vi "Button Config Pane.vi"(6 "_SubPanelMessages":refnum<notifier>, 9 "_myEmbeddedToFrameEvent":T6, 10 "_myEmbedded.Exit":refnum<user-event>, 11 "_Property Bundle":cluster{"Name":string, "Value":variant}[](array[cluster])) -> (1 "_Connection Informations":T1, 2 "_Scripter Input":T8)   [LabVIEW 2021]
doc: "Reads the value from the user button on the NI myRIO."
uses:
  <vilib>/myRIO/Common/Express VI Framework/typedefs/Config Pane to Framework Ref.ctl
  <vilib>/myRIO/Common/Express VI Framework/typedefs/Data Validate Ref.ctl
  <vilib>/myRIO/Common/Express VI Framework/typedefs/Scripter Input.ctl
  <vilib>/myRIO/Common/Express VI Framework/typedefs/WireThrough Terminal Names.ctl
  <vilib>/myRIO/Common/Express VI Framework/typedefs/Instrument Driver Method Descriptor Array.ctl
  <vilib>/myRIO/Common/Express VI Framework/typedefs/Instrument Driver Method Descriptor.ctl
  <vilib>/myRIO/Common/Express VI Framework/typedefs/Sub Panel Messages.ctl
  <vilib>/myRIO/Express VI/Onboard Devices/Button/Button Images.ctl
  <vilib>/myRIO/Common/Express VI Framework/typedefs/Connection Informations.ctl
  <vilib>/myRIO/Common/Instrument Driver Framework/Utilities/typedefs/Channel Types.ctl
panel:
  out "Description":string
  out "_Button Location":T2
  in  "_Terminal Name \n(Edit and make value default)":string[](array[string])=["Value"]
  in  "_Default Alias String":string
  in  "_VI Default Name (Edit and make value default)":string="Button"
  in  "Name:":string caption="Node name:"
  in  "_WireThrough Info (Edit and make value default)":T3={"WireThrough Top In"="DIO Ref In", "WireThrough Bottom In"="error in (no error)", "WireThrough Top Out"="DIO Ref Out", "WireThrough Bottom Out"="error out"}
  in  "_Template Array (Edit and make value default)":T4=[{"Function Name"="Smart Open", "VI Path"=path "<vilib>/myRIO/Instrument Drivers/Onboard IO/DIO/vis", "Script"=TRUE, "Inputs"=[{"name"="Channel Names", "value"=variant, "Config Pane Only"=TRUE, "Build Array"=FALSE, "Bundle Cluster"=FALSE, "Show Term"=FALSE, "alias"=[], "Required Input"=FALSE}], "Outputs"=[], "VI Class"=enum."Open", "Controls Refs[]"=[], "Inline"=FALSE}, {"Function Name"="Open", "VI Path"=path "<vilib>/myRIO/Instrument Drivers/Onboard IO/DIO/vis", "Script"=FALSE, "Inputs"=[], "Outputs"=[], "VI Class"=enum."Open", "Controls Refs[]"=[], "Inline"=FALSE}, {"Function Name"="Read", "VI Path"=path "<vilib>/myRIO/Instrument Drivers/Onboard IO/DIO/vis", "Script"=TRUE, "Inputs"=[], "Outputs"=[{"name"="Values", "value"=variant, "Show Term"=TRUE, "Index Array"=TRUE, "Unbundle Cluster"=FALSE, "alias"=["Button"]}], "VI Class"=enum."Data", "Controls Refs[]"=[], "Inline"=FALSE}, {"Function Name"="Write", "VI Path"=path "<vilib>/myRIO/Instrument Drivers/Onboard IO/DIO/vis", "Script"=FALSE, "Inputs"=[{"name"="Values", "value"=variant, "Config Pane Only"=FALSE, "Build Array"=TRUE, "Bundle Cluster"=FALSE, "Show Term"=TRUE, "alias"=[], "Required Input"=FALSE}], "Outputs"=[], "VI Class"=enum."Data", "Controls Refs[]"=[], "Inline"=FALSE}, {"Function Name"="Close", "VI Path"=path "<vilib>/myRIO/Instrument Drivers/Onboard IO/DIO/vis", "Script"=FALSE, "Inputs"=[], "Outputs"=[], "VI Class"=enum."Close", "Controls Refs[]"=[], "Inline"=FALSE}]
  in  "_Test Close":bool
  # "User Visible Area"
  # "NOTE: Tab Order has been set\nfor this Front Panel.\n\nSee Edit>>Set Tabbing Order...\n\nAll controls that are not visible at \nruntime are excluded from Tabbing order\n\n\nTo exlude a control from context\nhelp prefix its label text with a '-'"
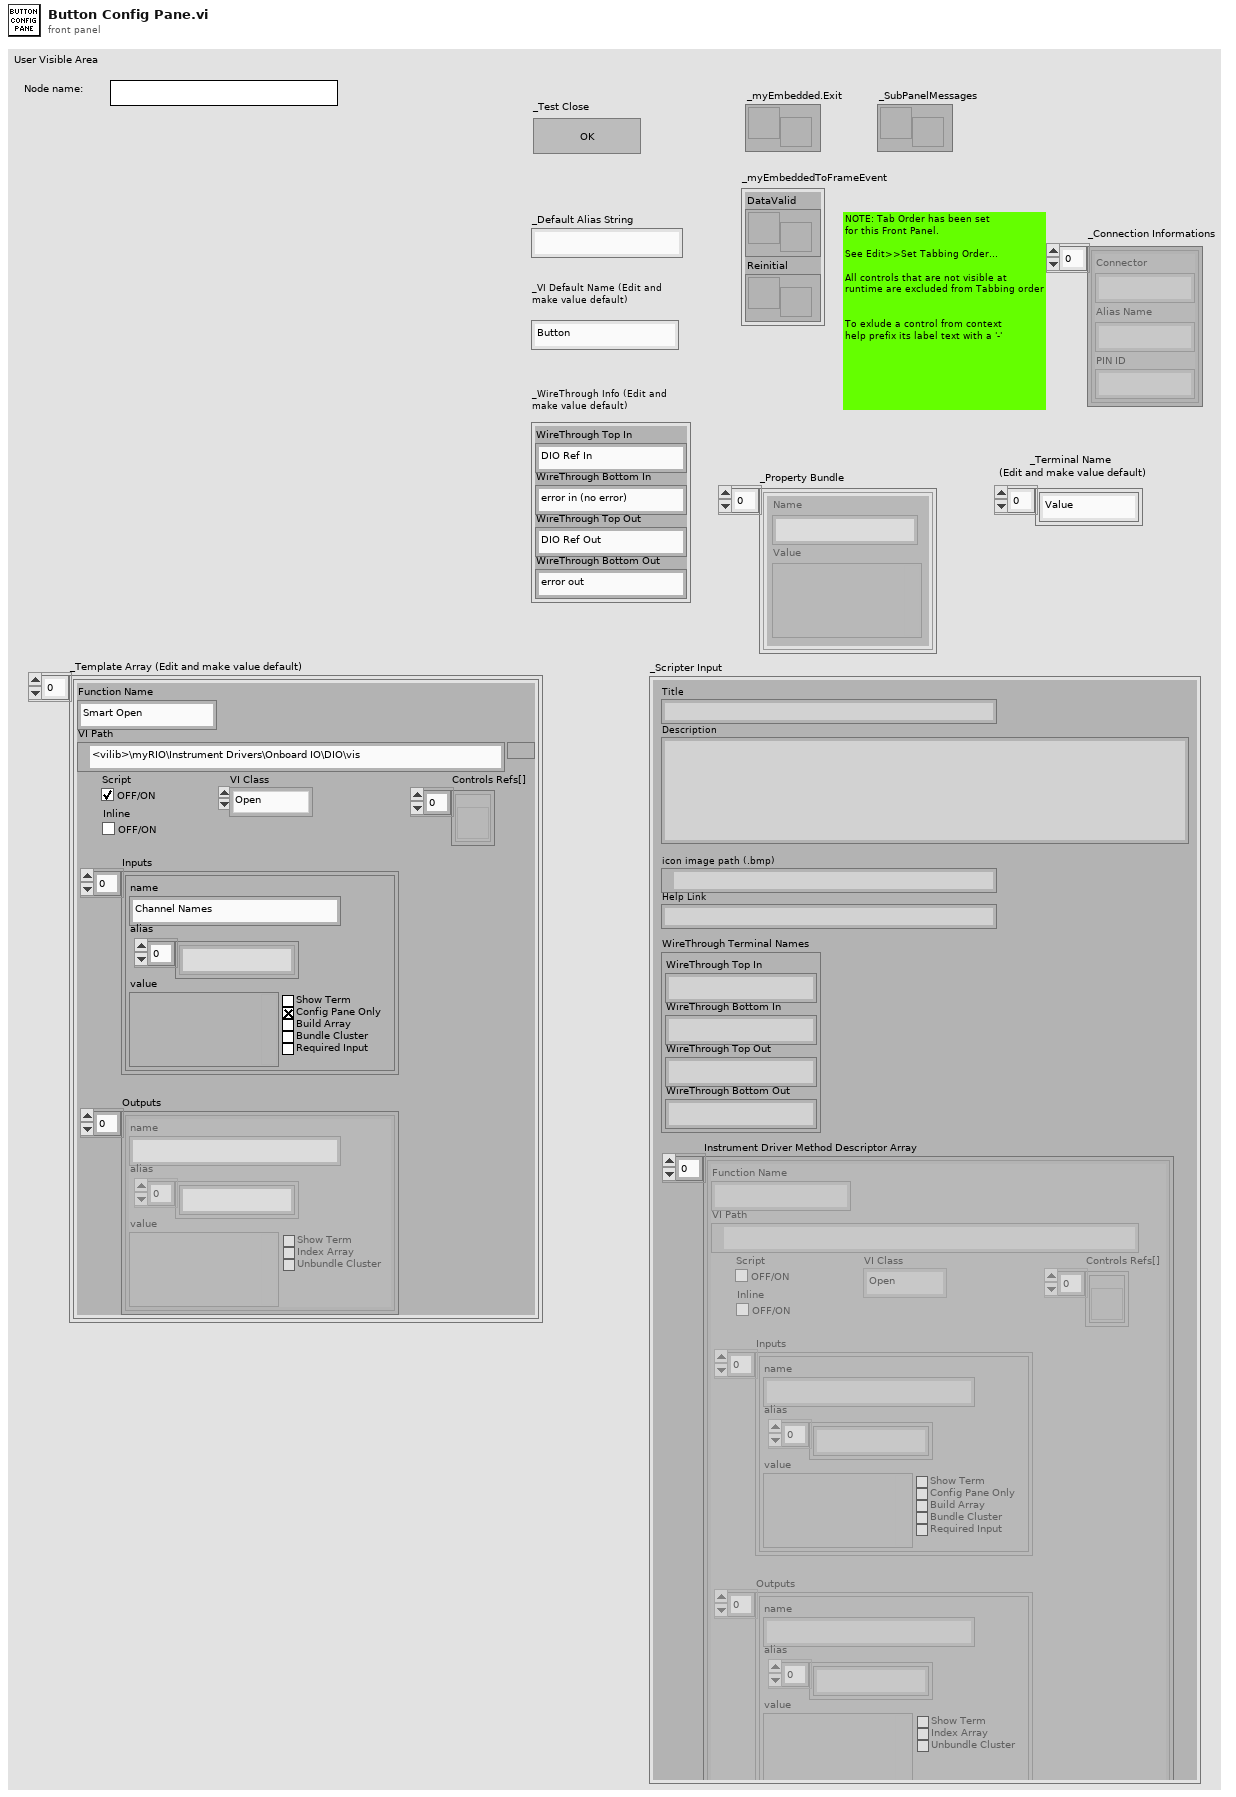
[diagram p1: front panel]
types:
  T1 = typedef "Connection Informations.ctl" = cluster{"Connector":string, "Alias Name":string, "PIN ID":string}[]
  T2 = typedef "Button Images.ctl" = u16
  T3 = typedef "WireThrough Terminal Names.ctl" = cluster{"WireThrough Top In":string, "WireThrough Bottom In":string, "WireThrough Top Out":string, "WireThrough Bottom Out":string}
  T4 = typedef "Instrument Driver Method Descriptor Array.ctl" = T5[]
  T5 = typedef "Instrument Driver Method Descriptor.ctl" = cluster{"Function Name":string, "VI Path":path, "Script":bool, "Inputs":cluster{"name":string, "value":variant, "Config Pane Only":bool, "Build Array":bool, "Bundle Cluster":bool, "Show Term":bool, "alias":string[], "Required Input":bool}[], "Outputs":cluster{"name":string, "value":variant, "Show Term":bool, "Index Array":bool, "Unbundle Cluster":bool, "alias":string[]}[], "VI Class":enum16{"Open", "Configure", "Data", "Manage", "Close"}, "Controls Refs[]":refnum<vi>[], "Inline":bool}
  T6 = typedef "Config Pane to Framework Ref.ctl" = cluster{"DataValid":T7, "Reinitial":refnum<user-event>}
  T7 = typedef "Data Validate Ref.ctl" = refnum<user-event>
  T8 = typedef "Scripter Input.ctl" = cluster{"Title":string, "Description":string, "icon image path (.bmp)":path, "Help Link":string, "WireThrough Terminal Names":T3, "Instrument Driver Method Descriptor Array":T4}
  T9 = typedef "Channel Types.ctl" = enum32{"Unknown", "AI", "AO", "DIO - DI", "DIO", "DIO - DO", "I2C", "PWM", "Encoder", "SPI", "UART", "Accelerometer", "DIO - LED", "DIO - Button", "AI (N Samples)", "AudioIn (N Samples)", "AO (N Samples)", "AudioOut (N Samples)", "DI (N Samples)", "DO (N Samples)", "AI IRQ", "DI IRQ", "Timer IRQ", "RSL", "Relay", "CAN", "AI (Continuous)", "AO (Continuous)"}
  T10 = typedef "Sub Panel Messages.ctl" = enum16{"Initialized"}
  T11 = typedef "Channel Info.ctl" = cluster{"Channel Name":string, "Alias":string, "Used?":bool, "Not Support?":bool, "Property Bundle":cluster{"Name":string, "Value":variant}[]}
  T12 = cluster{"name":string, "value":variant, "Config Pane Only":bool, "Build Array":bool, "Bundle Cluster":bool, "Show Term":bool, "alias":string[], "Required Input":bool}[]
  T13 = cluster{"name":string, "value":variant, "Config Pane Only":bool, "Build Array":bool, "Bundle Cluster":bool, "Show Term":bool, "alias":string[], "Required Input":bool}
  T14 = cluster{"name":string, "value":variant, "Show Term":bool, "Index Array":bool, "Unbundle Cluster":bool, "alias":string[]}[]
  T15 = cluster{"name":string, "value":variant, "Show Term":bool, "Index Array":bool, "Unbundle Cluster":bool, "alias":string[]}
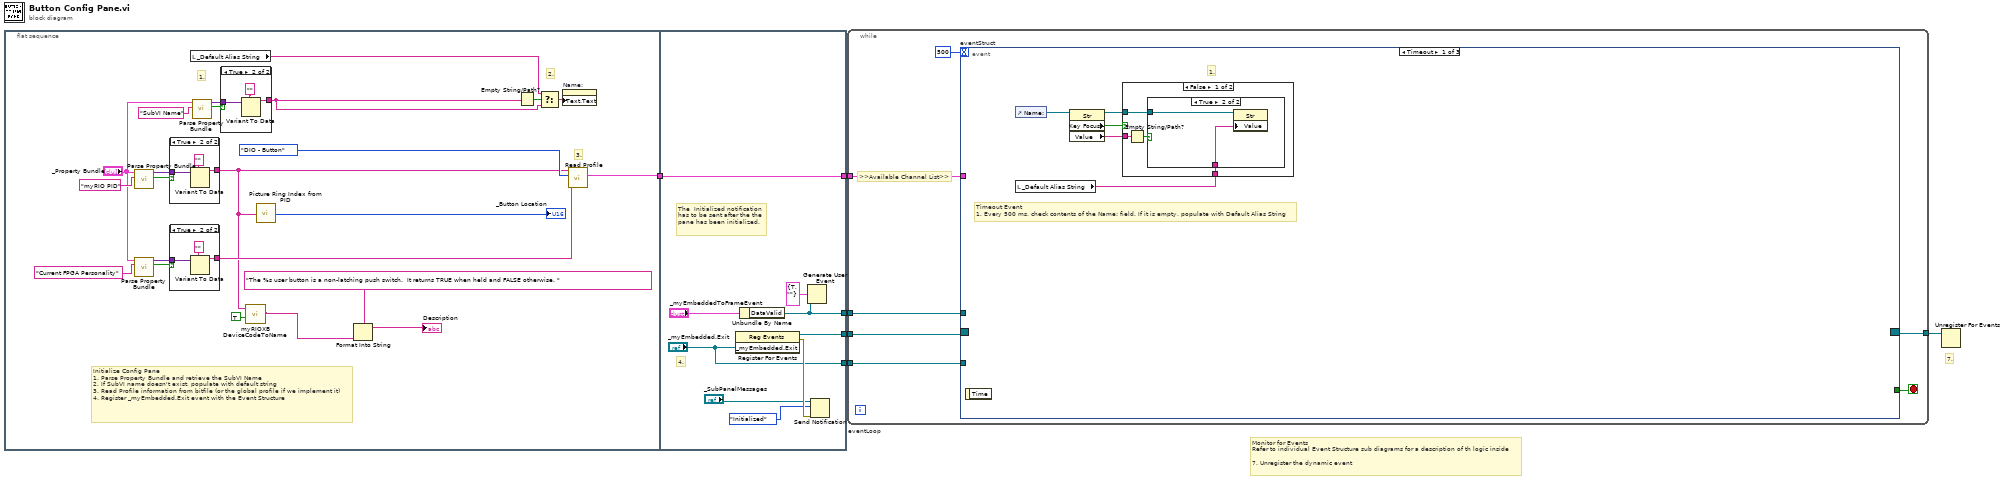
[diagram p0: block diagram]
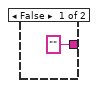
[diagram p2: hidden frame]
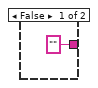
[diagram p3: hidden frame]
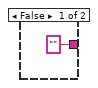
[diagram p4: hidden frame]
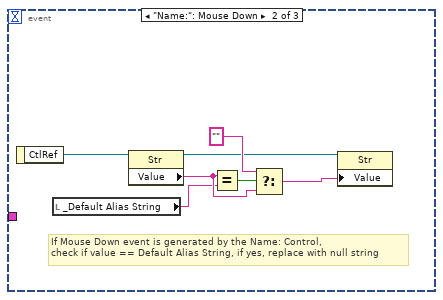
[diagram p7: hidden frame]
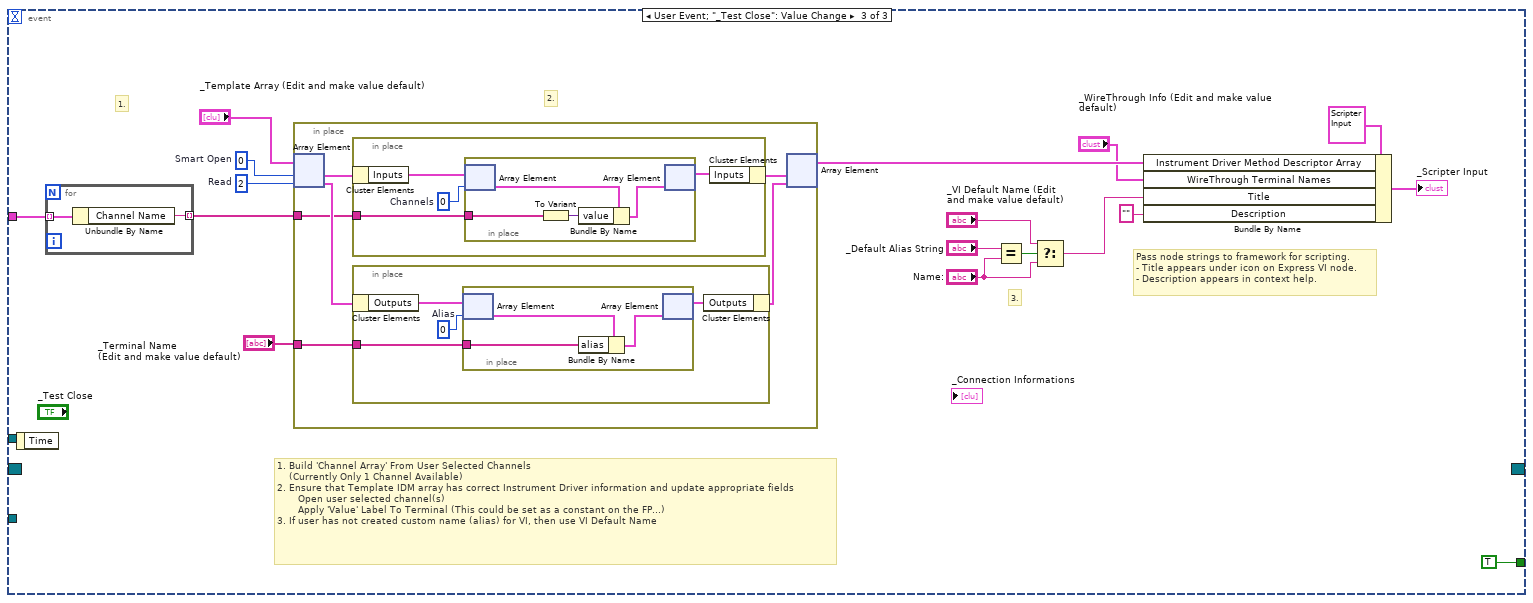
[diagram p8: hidden frame]
diagram:
  # "7."
  # "Monitor for Events\nRefer to individual Event Structure sub diagrams for a description of th logic inside\n\n7. Unregister the dynamic event"
  n1 = flat-sequence {
    tunnel: [w29] -> w4
    tunnel: [w50] -> w5
    tunnel: w4 -> [w50]
    tunnel: [w43] -> w3
    tunnel: [w45] -> w2
    tunnel: ["_myEmbedded.Exit"] -> w1
    frame #0 {
      # "3."
      # "1."
      # "2."
      # "Initialize Config Pane\n1. Parse Property Bundle and retrieve the SubVI Name\n2. If SubVI name doesn't exist, populate with default string\n3. Read Profile information from bitfile (or the global profile if we implement it)\n4. Register _myEmbedded.Exit event with the Event Structure"
      n2 = call <vilib>:"Parse Property Bundle.vi"("Name"="myRIO PID", "Property Bundle"="_Property Bundle") -> ("Found?"=w28:bool, "Value"=w27:variant)  [unwired: 8 in]
      n3 = call <vilib>:"Parse Property Bundle.vi"("Name"="Current FPGA Personality", "Property Bundle"="_Property Bundle") -> ("Found?"=w14:bool, "Value"=w15:variant)  [unwired: 8 in]
      n4 = case shown="True" w28 {
        tunnel: w27 -> [_ w41]
        tunnel: ["" ("Name") w39] -> w11
        frame False {
        }
        frame True {
          n5 = Variant To Data(type="" ("Name"), Variant=w41) -> (data=w39:string)  [unwired: 1 in, 1 out]
        }
      }
      n6 = case shown="True" w14 {
        tunnel: w15 -> [_ w33]
        tunnel: ["" ("Name") w31] -> w13
        frame False {
        }
        frame True {
          n7 = Variant To Data(type="" ("Name"), Variant=w33) -> (data=w31:string)  [unwired: 1 in, 1 out]
        }
      }
      n8 = local read "_Default Alias String"() -> (w22:string)
      n9 = call <vilib>:"Parse Property Bundle.vi"("Name"="SubVI Name", "Property Bundle"="_Property Bundle") -> ("Found?"=w20:bool, "Value"=w19:variant)  [unwired: 8 in]
      n10 = case shown="True" w20 {
        tunnel: w19 -> [_ w37]
        tunnel: ["" ("Name") w35] -> w18
        frame False {
        }
        frame True {
          n11 = Variant To Data(type="" ("Name"), Variant=w37) -> (data=w35:string)  [unwired: 1 in, 1 out]
        }
      }
      n12 = call <vilib>:"myRIOXB DeviceCodeToName.vi"("FullName?"=TRUE, "Device Code"=w11) -> ("Name"=w9:string)  [unwired: 9 in]
      n13 = call <vilib>:"Picture Ring Index from PID.vi"("myRIO PID"=w11) -> ("picture ring index"=→"_Button Location":u32)
      n14 = Format Into String(format string="The %s user button is a non-latching push switch.  It returns TRUE when held and FALSE otherwise. ", w9) -> (resulting string=→"Description":string)  [unwired: 2 in, 1 out]
      n15 = Empty String/Path?(string/path=w18) -> (empty?=w24:bool)
      n16 = Select(t=w22, s=w24, f=w18) -> (s? t:f=w23:string)
      n17 = property on="Name:" class="Str"("Text.Text"=w23) -> ()  [unwired: 2 in, 2 out]
      n18 = call <vilib>:"Read Profile.vi"("FPGA Name"=w13, "Channel to Read"=Channel_Types."DIO - Button", "myRIO PID"=w11) -> ("Channel List Out"=w29:T11[])  [unwired: 7 in, 1 out]
    }
    frame #1 {
      # "The  Initialized notification has to be sent after the the pane has been initialized."
      # "4."
      n19 = register-events("_myEmbedded.Exit") -> (reference out=w45:refnum<event-registration>, error out=w49:errorcluster)  [unwired: 2 in]
      n20 = Unbundle By Name("_myEmbeddedToFrameEvent") -> ("DataValid"=w43:T7)
      n21 = Generate User Event(user event=w43, event data cluster=cluster{"Valid":bool, "Invalid Info":string} {"Valid"=TRUE, "Invalid Info"=""} ("event data")) -> ()  [unwired: 2 in, 2 out]
      n22 = Send Notification(notification=Sub_Panel_Messages."Initialized", notifier="_SubPanelMessages", error in (no error)=w49) -> ()  [unwired: 2 out]
    }
  }
  n23 = while "eventLoop" {
    tunnel: w2 -> [w56]
    tunnel: [w55] -> w6
    tunnel: w3 -> [w52]
    tunnel: w5 -> [w51]
    tunnel: w1 -> [w53]
    stop <- w57 stop-if-true
    # ">>Available Channel List>>"
    n24 = event "eventStruct" shown="[0] Timeout" {
      selector: w56 -> [_ _ _]
      dyn-events: [_ _ _] -> w55
      timeout: 500 -> [_ _ _]
      tunnel: [_ _ TRUE ("_Test Close")] -> w57
      tunnel: w51 -> [_ _ w78]
      tunnel: w53 -> [_ _ _]
      tunnel: w52 -> [_ _ _]
      event Timeout {
        # "Timeout Event\n1. Every 500 ms, check contents of the Name: field. If it is empty, populate with Default Alias String"
        # "1."
        n25 = event-data() -> ()  [unwired: 1 in, 1 out]
        n26 = control-ref of="Name:"() -> (w60:refnum<vi>)
        n27 = local read "_Default Alias String"() -> (w58:string)
        n28 = property on="Property Node" class="Str"(reference=w60) -> (reference out=w59:refnum<vi>, "Key Focus"=w61:bool, "Value"=w62:string)  [unwired: 1 in, 1 out]
        n29 = case shown="False" w61 {
          tunnel: w62 -> [w66 _]
          tunnel: w59 -> [w64 _]
          tunnel: w58 -> [w63 _]
          frame False {
            n30 = Empty String/Path?(string/path=w66) -> (empty?=w65:bool)
            n31 = case shown="True" w65 {
              tunnel: w64 -> [_ w68]
              tunnel: w63 -> [_ w67]
              frame False {
              }
              frame True {
                n32 = property on="Property Node" class="Str"(reference=w68, "Value"=w67) -> ()  [unwired: 1 in, 2 out]
              }
            }
          }
          frame True {
          }
        }
      }
      event "Name:": Mouse Down {
        # "If Mouse Down event is generated by the Name: Control,\ncheck if value == Default Alias String, if yes, replace with null string"
        n33 = event-data() -> ("CtlRef"=w75:refnum<vi>)  [unwired: 1 in]
        n34 = local read "_Default Alias String"() -> (w69:string)
        n35 = property class="Str"(reference=w75) -> (reference out=w71:refnum<vi>, "Value"=w70:string)  [unwired: 1 in, 1 out]
        n36 = Equal?(x=w70, y=w69) -> (x = y?=w74:bool)
        n37 = Select(t="", s=w74, f=w70) -> (s? t:f=w72:string)
        n38 = property class="Str"(reference=w71, "Value"=w72) -> ()  [unwired: 1 in, 2 out]
      }
      event User Event; "_Test Close": Value Change {
        w79 = 2  # Read
        w89 = 0  # Smart Open
        # "2."
        # "1."
        # "1. Build 'Channel Array' From User Selected Channels \n    (Currently Only 1 Channel Available)\n2. Ensure that Template IDM array has correct Instrument Driver information and update appropriate fields\n       Open user selected channel(s)\n       Apply 'Value' Label To Terminal (This could be set as a constant on the FP...)\n3. If user has not created custom name (alias) for VI, then use VI Default Name"
        # "3."
        # "Pass node strings to framework for scripting.\n- Title appears under icon on Express VI node.\n- Description appears in context help."
        n39 = event-data() -> ()  [unwired: 1 in, 1 out]
        n40 = for {
          tunnel: w78 -> [w94] mode=indexing
          tunnel: [w93] -> w77 mode=indexing
          n41 = Unbundle By Name(w94) -> ("Channel Name"=w93:string)
        }
        n42 = in-place {
          in-place-border: w77 -> [w96]
          in-place-border: "_Terminal Name \n(Edit and make value default)" -> [w95]
          n43 = in-place-array #1("_Template Array (Edit and make value default)", w89, w79) -> (w100:T5, w98:T5)
          n44 = in-place {
            in-place-border: w96 -> [w108]
            w109 = 0  # Channels
            n45 = in-place-cluster #2(w100) -> ("Inputs"=w111:T12)
            n46 = in-place {
              in-place-border: w108 -> [w112]
              n47 = in-place-array #3(w111, w109) -> (w115:T13)
              n48 = To Variant(anything=w112) -> (Variant=w113:variant)
              n49 = Bundle By Name(cluster=w115, "value"=w113) -> (w114:T13)
              n50 = in-place-array #3(w114) -> (w110:T12)  [unwired: 1 out]
            }
            n51 = in-place-cluster #2("Inputs"=w110) -> (w99:T5)
          }
          n52 = in-place {
            in-place-border: w95 -> [w101]
            w104 = 0  # Alias
            n53 = in-place-cluster #4(w98) -> ("Outputs"=w103:T14)
            n54 = in-place {
              in-place-border: w101 -> [w105]
              n55 = in-place-array #5(w103, w104) -> (w107:T15)
              n56 = Bundle By Name(cluster=w107, "alias"=w105) -> (w106:T15)
              n57 = in-place-array #5(w106) -> (w102:T14)  [unwired: 1 out]
            }
            n58 = in-place-cluster #4("Outputs"=w102) -> (w97:T5)
          }
          n59 = in-place-array #1(w99, w97) -> (w91:T4)  [unwired: 2 out]
        }
        n60 = Equal?(x="_Default Alias String", y="Name:") -> (x = y?=w83:bool)
        n61 = Select(t="_VI Default Name (Edit and make value default)", s=w83, f="Name:") -> (s? t:f=w82:string)
        n62 = Bundle By Name(cluster=T8 {"Title"="", "Description"="", "icon image path (.bmp)"=path "", "Help Link"="", "WireThrough Terminal Names"={"WireThrough Top In"="", "WireThrough Bottom In"="", "WireThrough Top Out"="", "WireThrough Bottom Out"=""}, "Instrument Driver Method Descriptor Array"=[]} ("Scripter Input"), "Instrument Driver Method Descriptor Array"=w91, "WireThrough Terminal Names"="_WireThrough Info (Edit and make value default)", "Title"=w82, "Description"="" ("Title")) -> (→"_Scripter Input":T8)
      }
    }
  }
  n63 = Unregister For Events(event registration refnum=w6) -> ()  [unwired: 1 in, 1 out]
